vi "Manual Assembly old.vi"() -> ()   [LabVIEW 2021]
uses:
  Classes/Routine/Routine Enum.ctl
  Classes/Routine/TypeOfHexaboard.ctl
  Classes/Assembly/Assembly Run.lvclass
  Classes/Workspace/Fixture Enum.ctl
  Classes/Controller/Controller.lvclass
  Classes/Workspace/Fixture.lvclass
  Classes/Routine/Routine.lvclass
panel:
  in  "Submit":bool
  out "Type of Hexaboard Confirmation":T1
  in  "Type of Component":T1
  in  "Update":bool
  in  "Stage":i32(listbox)=-1
  in  "Routine":T2=enum."Dispense on Plate"
  in  "Stop":bool
  in  "Remove":bool
  in  "Add":bool
  in  "Go":bool
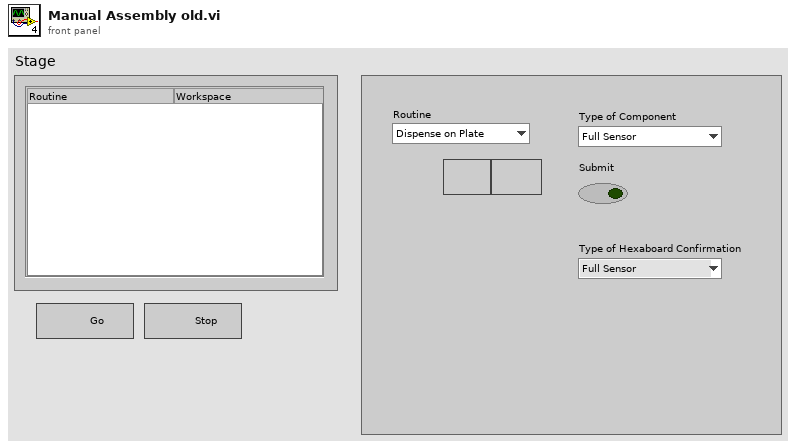
[diagram p1: front panel]
types:
  T1 = typedef "Routine.lvclass/TypeOfHexaboard.ctl" = enum16{"Full Sensor", "Full PCB", "Right Partial PCB", "Right Partial Sensor", "Al Dummy Right Partial Sensor"}
  T2 = typedef "Routine.lvclass/Routine Enum.ctl" = enum16{"Primary Pick Up", "Secondary Pick Up", "Put Down All", "Secure Syringe", "Release Syringe", "Dispense on Plate", "Dispense on Sensor", "Pick Up All", "Put Down Secondary", "Dispense on Kapton", "Full Assembly"}
  T3 = typedef "Controller.lvclass/Controllers.ctl" = cluster{"I-O.lvclass":refnum<class "I-O.lvclass">, "Gantry":refnum<k24>, "Dispenser":refnum<visa-resource-name>}
  T4 = typedef "Fixture.lvclass/Fixture Enum.ctl" = enum16{"Assembly Tray", "Syringe Space", "Component", "Pick Up Tool", "Current Position"}
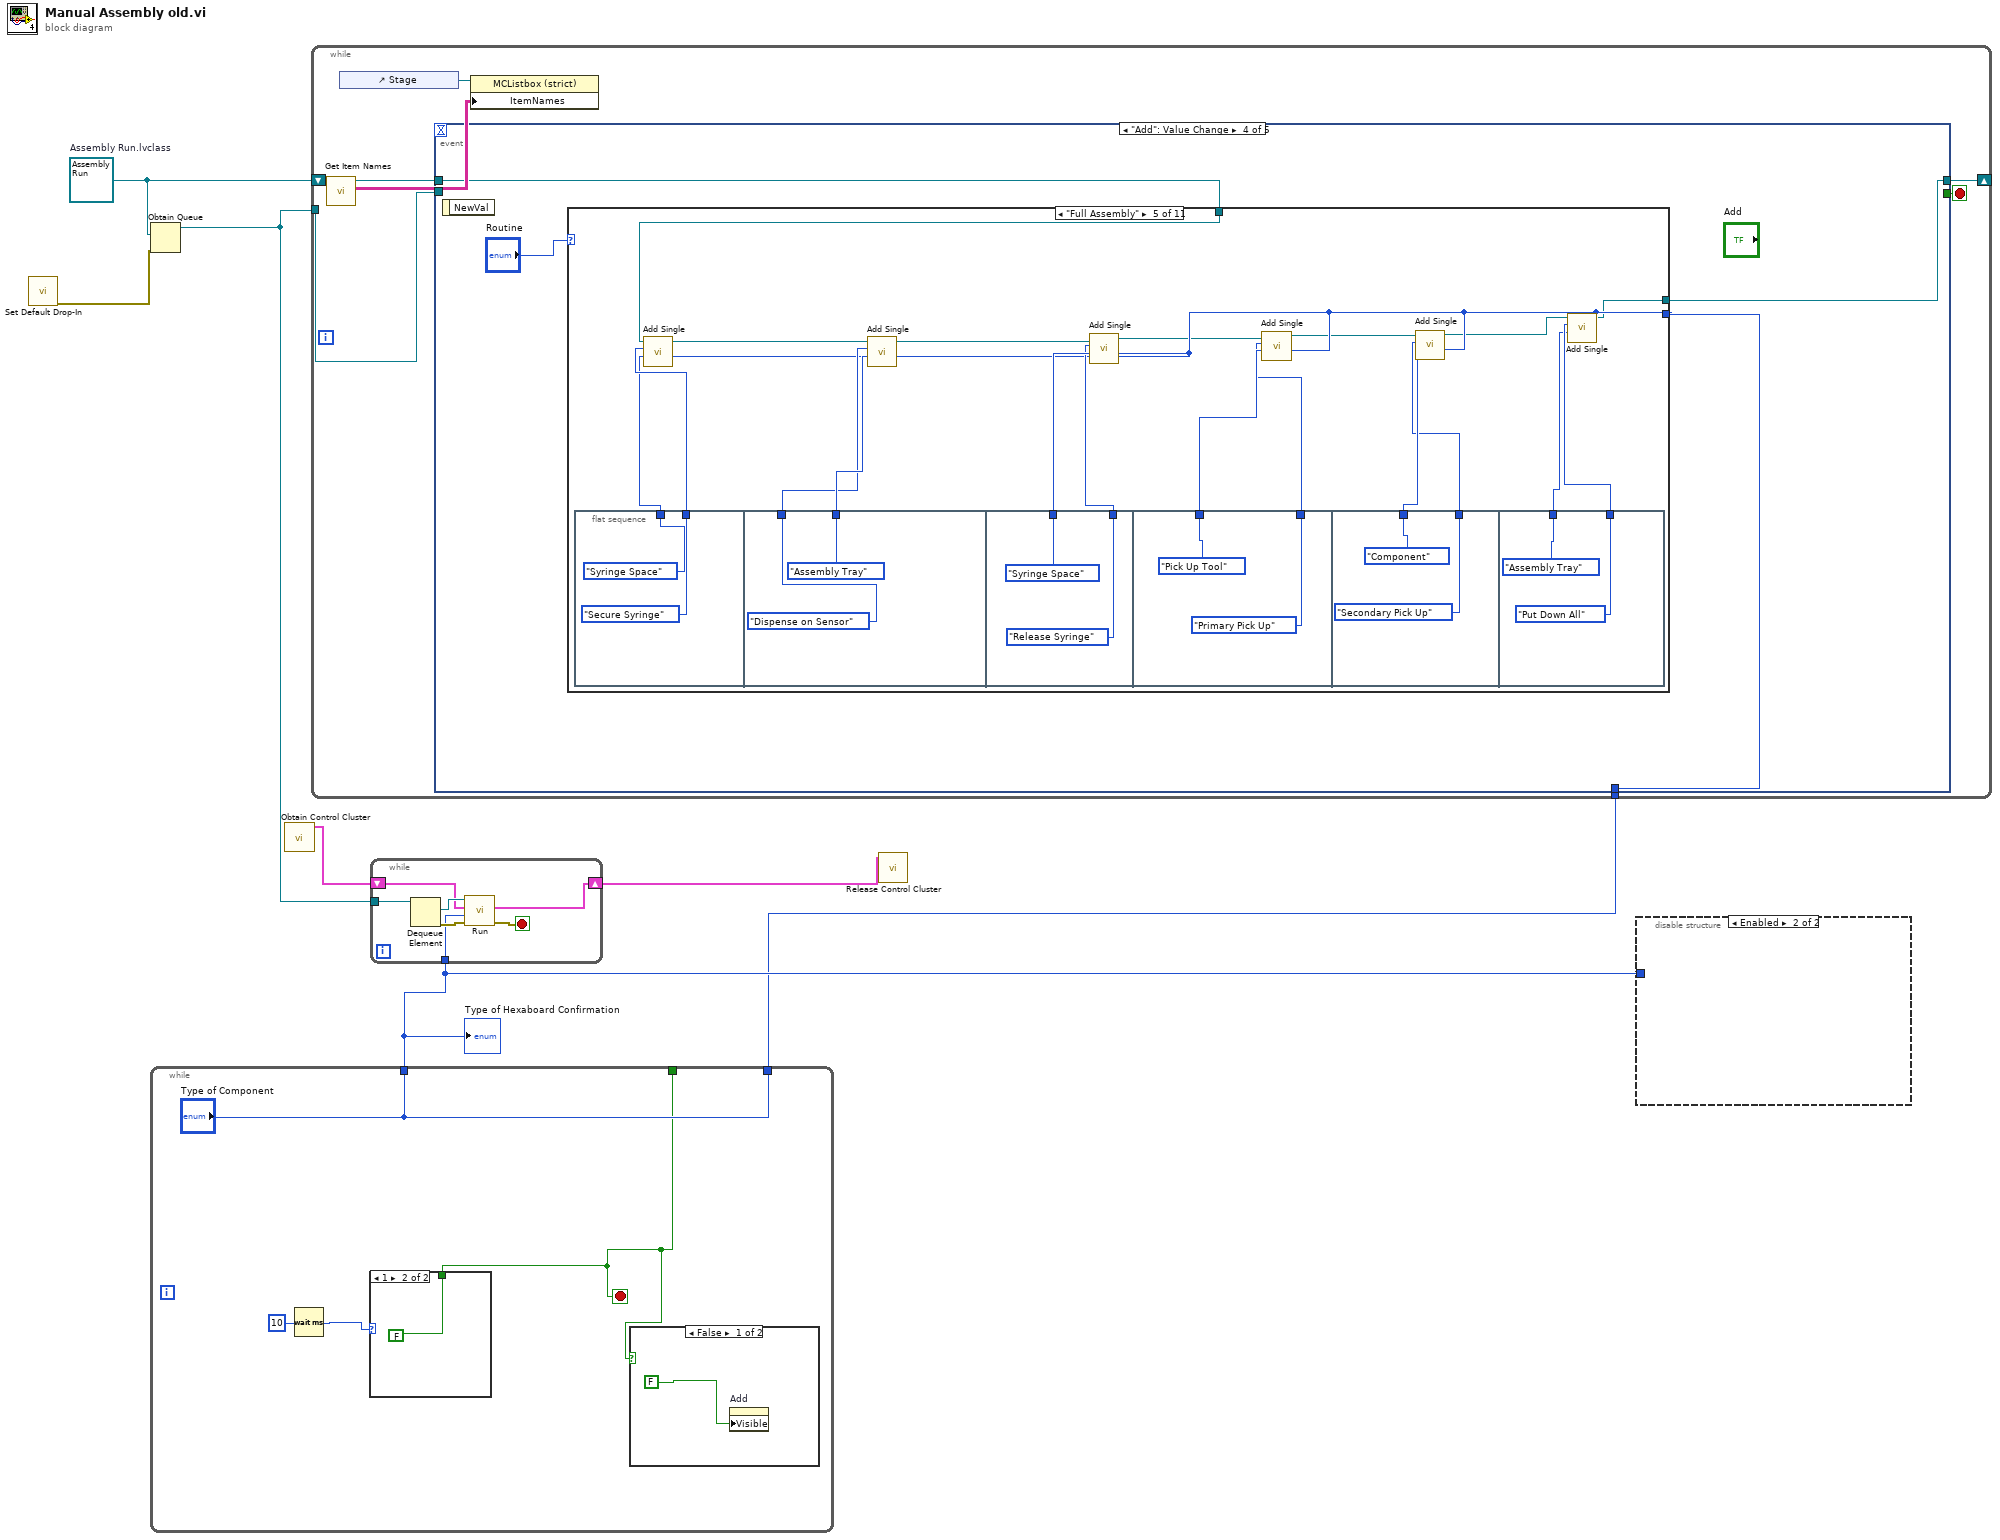
[diagram p0: block diagram]
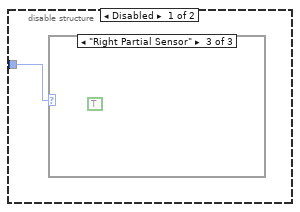
[diagram p2: hidden frame]
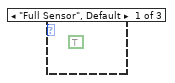
[diagram p3: hidden frame]
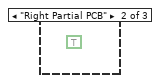
[diagram p4: hidden frame]
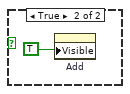
[diagram p5: hidden frame]
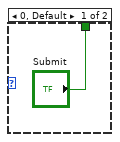
[diagram p6: hidden frame]
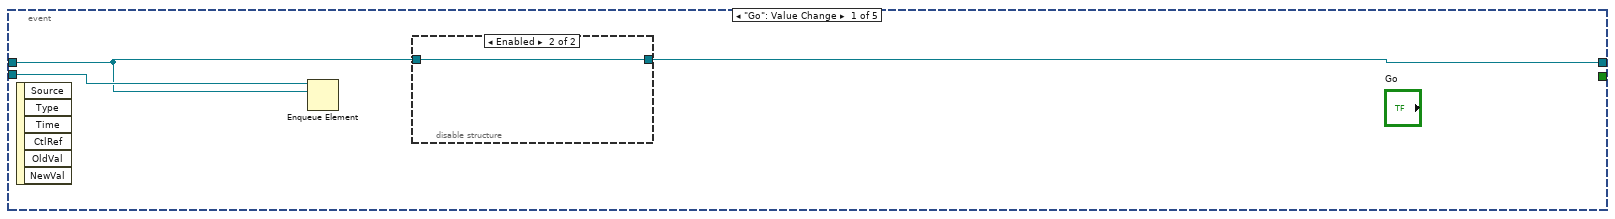
[diagram p7: hidden frame]
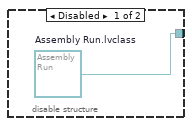
[diagram p8: hidden frame]
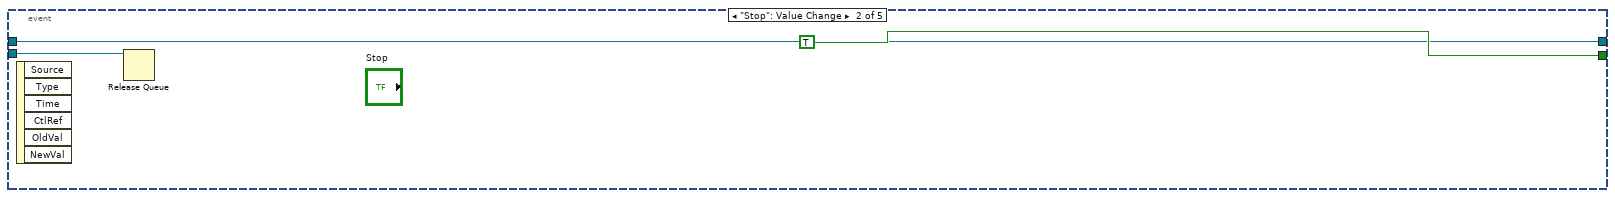
[diagram p9: hidden frame]
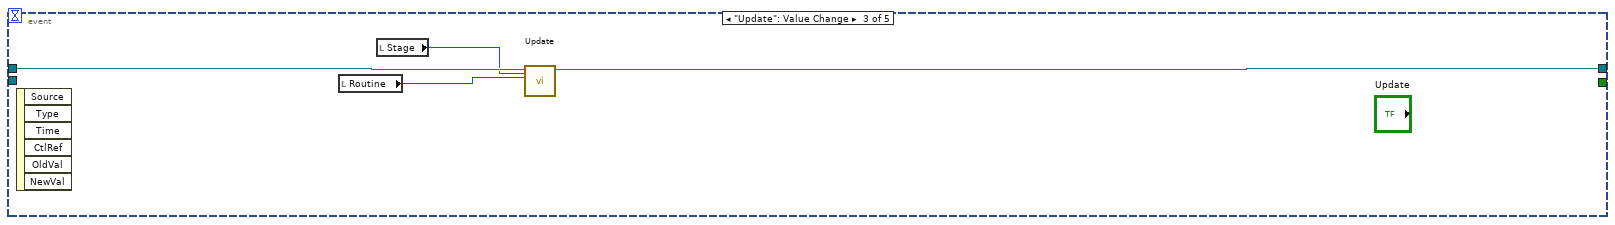
[diagram p10: hidden frame]
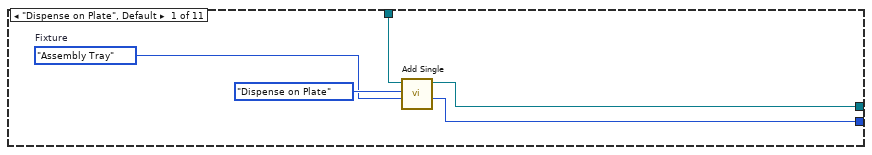
[diagram p11: hidden frame]
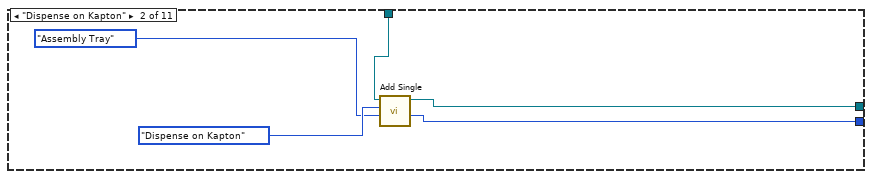
[diagram p12: hidden frame]
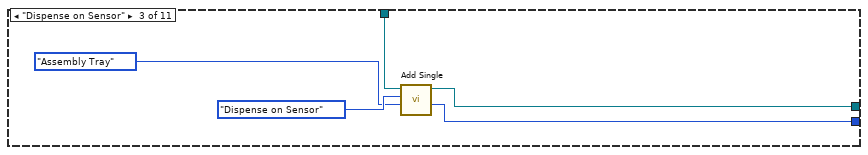
[diagram p13: hidden frame]
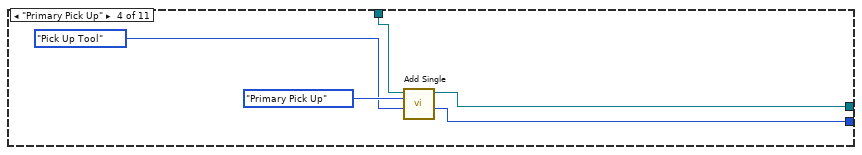
[diagram p14: hidden frame]
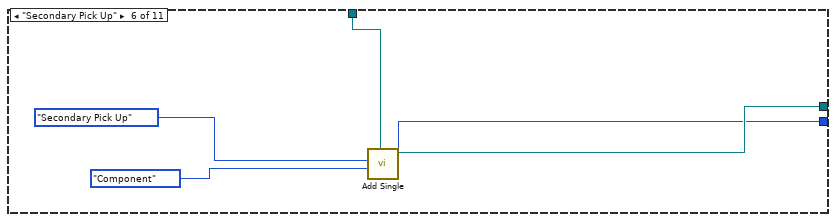
[diagram p15: hidden frame]
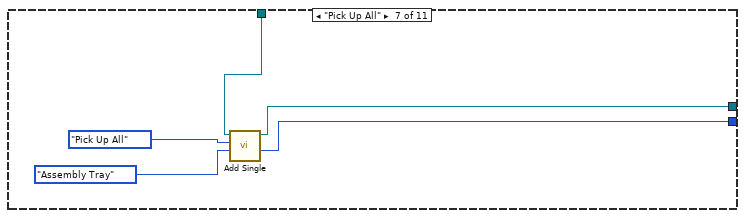
[diagram p16: hidden frame]
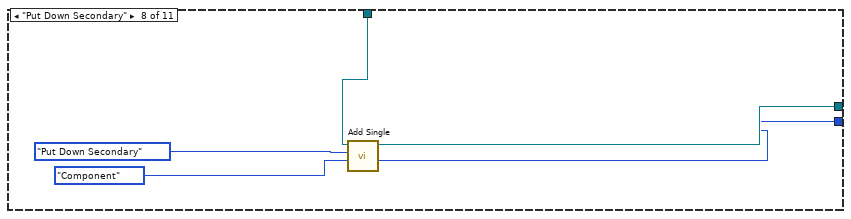
[diagram p17: hidden frame]
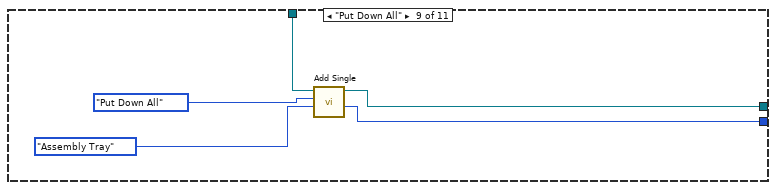
[diagram p18: hidden frame]
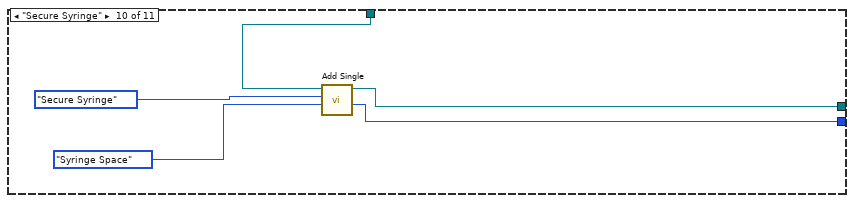
[diagram p19: hidden frame]
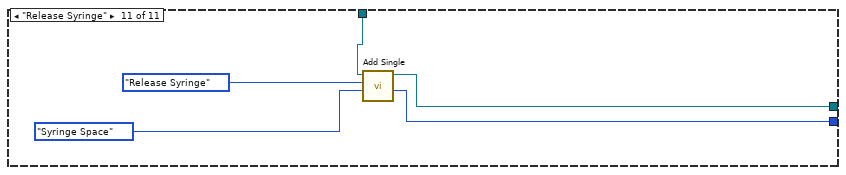
[diagram p20: hidden frame]
diagram:
  w3 = refnum<class "Assembly Run.lvclass"> refnum  # Assembly Run.lvclass
  n1 = call "Set Default Drop-In.vi"() -> ("error out"=w5:errorcluster)  [unwired: 11 in]
  n2 = Obtain Queue(element data type=w3, error in (no error)=w5) -> (queue out=w7:refnum<queue>)  [unwired: 3 in, 2 out]
  n3 = while {
    tunnel: ["Type of Component"] -> w2
    tunnel: ["Type of Component"] -> w1
    tunnel: [w8] -> _
    stop <- w8 stop-if-true
    n4 = Wait (ms)(milliseconds to wait=u32 10) -> (millisecond timer value=w10:u32)
    n5 = case shown="1" w10 {
      tunnel: ["Submit" FALSE] -> w8
      frame 0, Default {
      }
      frame 1 {
      }
    }
    n6 = case shown="False" w8 {
      frame False {
        n7 = property on="Add" class="Bool"("Visible"=FALSE) -> ()  [unwired: 2 in, 2 out]
      }
      frame True {
        n8 = property on="Add" class="Bool"("Visible"=TRUE) -> ()  [unwired: 2 in, 2 out]
      }
    }
  }
  "Type of Hexaboard Confirmation" <- w2
  n9 = call "Obtain Control Cluster.vi"() -> ("Control Out"=w4:T3)  [unwired: 11 in]
  n10 = while {
    shift-right: [w17] -> _
    shift-left: w3 -> [w19]
    tunnel: w7 -> [w22]
    tunnel: w1 -> [w16]
    stop <- w23 stop-if-true
    n11 = call "Get Item Names.vi"("Assembly Run in"=w19) -> ("Item names"=w21:string[][], "Assembly Run out"=w18:refnum<class "Assembly Run.lvclass">)  [unwired: 8 in, 1 out]
    n12 = control-ref of="Stage"() -> (w20:refnum<vi>)
    n13 = event shown="[3] \"Add\": Value Change" {
      selector: _ -> [_ _ _ _ _]
      dyn-events: _ -> [_ _ _ _ _]
      timeout: _ -> [_ _ _ _ _]
      tunnel: [_ TRUE _ _ _] -> w23
      tunnel: w18 -> [w24 w30 w35 w37 w124]
      tunnel: [w25 w30 w34 w36 w123] -> w17
      tunnel: w22 -> [w26 w29 _ _ _]
      tunnel: w16 -> [_ _ _ w38 _]
      event "Go": Value Change {
        n14 = event-data() -> ()  [unwired: 1 in, 6 out]
        n15 = Enqueue Element(queue=w26, element=w24) -> ()  [unwired: 2 in, 3 out]
        n16 = disable-structure shown="Enabled" {
          disable-tunnel: [w27 w28] -> w25
          disable-tunnel: w24 -> [_ w28]
          frame Disabled {
            w27 = refnum<class "Assembly Run.lvclass"> refnum  # Assembly Run.lvclass
          }
          frame Enabled {
          }
        }
      }
      event "Stop": Value Change {
        n17 = event-data() -> ()  [unwired: 1 in, 6 out]
        n18 = Release Queue(queue=w29) -> ()  [unwired: 2 in, 3 out]
      }
      event "Update": Value Change {
        n19 = event-data() -> ()  [unwired: 1 in, 6 out]
        n20 = local read "Routine"() -> (w33:T2)
        n21 = local read "Stage"() -> (w32:i32)
        n22 = call "Update.vi"("Row"=w32, "Routine"=w33, "Assembly Run in"=w35) -> ("Assembly Run out"=w34:refnum<class "Assembly Run.lvclass">)  [unwired: 7 in, 1 out]
      }
      event "Add": Value Change {
        n23 = event-data() -> ()  [unwired: 1 in, 1 out]
        n24 = case shown="\"Full Assembly\"" "Routine" {
          tunnel: w38 -> [w40 w47 w50 w55 w66 w92 w99 w102 w109 w114 w119]
          tunnel: w37 -> [w42 w45 w52 w56 w77 w94 w97 w103 w107 w112 w117]
          tunnel: [w41 w46 w51 w57 w60 w93 w98 w106 w108 w113 w118] -> w36
          frame "Dispense on Plate", Default {
            w43 = Fixture_Enum."Assembly Tray"  # Fixture
            n25 = call-dynamic "Add Single.vi"("Type of Hexaboard"=w40, "Fixture"=w43, "Routine"=Routine_Enum."Dispense on Plate", "UI in"=w42) -> ("UI out"=w41:refnum<class "Assembly Run.lvclass">)  [unwired: 5 in, 1 out]
          }
          frame "Dispense on Kapton" {
            n26 = call-dynamic "Add Single.vi"("Type of Hexaboard"=w47, "Fixture"=Fixture_Enum."Assembly Tray", "Routine"=Routine_Enum."Dispense on Kapton", "UI in"=w45) -> ("UI out"=w46:refnum<class "Assembly Run.lvclass">)  [unwired: 5 in, 1 out]
          }
          frame "Dispense on Sensor" {
            n27 = call-dynamic "Add Single.vi"("Type of Hexaboard"=w50, "Fixture"=Fixture_Enum."Assembly Tray", "Routine"=Routine_Enum."Dispense on Sensor", "UI in"=w52) -> ("UI out"=w51:refnum<class "Assembly Run.lvclass">)  [unwired: 5 in, 1 out]
          }
          frame "Primary Pick Up" {
            n28 = call-dynamic "Add Single.vi"("Type of Hexaboard"=w55, "Fixture"=Fixture_Enum."Pick Up Tool", "Routine"=Routine_Enum."Primary Pick Up", "UI in"=w56) -> ("UI out"=w57:refnum<class "Assembly Run.lvclass">)  [unwired: 5 in, 1 out]
          }
          frame "Full Assembly" {
            n29 = flat-sequence {
              tunnel: [Routine_Enum."Secure Syringe" ("Routine")] -> w79
              tunnel: [Fixture_Enum."Syringe Space" ("Fixture")] -> w78
              tunnel: [Fixture_Enum."Assembly Tray" ("Fixture")] -> w75
              tunnel: [Routine_Enum."Dispense on Sensor" ("Routine")] -> w74
              tunnel: [Fixture_Enum."Syringe Space" ("Fixture")] -> w73
              tunnel: [Routine_Enum."Release Syringe" ("Routine")] -> w72
              tunnel: [Fixture_Enum."Pick Up Tool" ("Fixture")] -> w71
              tunnel: [Routine_Enum."Primary Pick Up" ("Routine")] -> w70
              tunnel: [Fixture_Enum."Component" ("Fixture")] -> w69
              tunnel: [Routine_Enum."Secondary Pick Up" ("Routine")] -> w68
              tunnel: [Routine_Enum."Put Down All" ("Routine")] -> w67
              tunnel: [Fixture_Enum."Assembly Tray" ("Fixture")] -> w65
              frame #0 {
              }
              frame #1 {
              }
              frame #2 {
              }
              frame #3 {
              }
              frame #4 {
              }
              frame #5 {
              }
            }
            n30 = call-dynamic "Add Single.vi"("Type of Hexaboard"=w66, "Fixture"=w78, "Routine"=w79, "UI in"=w77) -> ("UI out"=w76:refnum<class "Assembly Run.lvclass">)  [unwired: 5 in, 1 out]
            n31 = call-dynamic "Add Single.vi"("Type of Hexaboard"=w66, "Fixture"=w75, "Routine"=w74, "UI in"=w76) -> ("UI out"=w64:refnum<class "Assembly Run.lvclass">)  [unwired: 5 in, 1 out]
            n32 = call-dynamic "Add Single.vi"("Type of Hexaboard"=w66, "Fixture"=w73, "Routine"=w72, "UI in"=w64) -> ("UI out"=w63:refnum<class "Assembly Run.lvclass">)  [unwired: 5 in, 1 out]
            n33 = call-dynamic "Add Single.vi"("Type of Hexaboard"=w66, "Fixture"=w71, "Routine"=w70, "UI in"=w63) -> ("UI out"=w62:refnum<class "Assembly Run.lvclass">)  [unwired: 5 in, 1 out]
            n34 = call-dynamic "Add Single.vi"("Type of Hexaboard"=w66, "Fixture"=w69, "Routine"=w68, "UI in"=w62) -> ("UI out"=w61:refnum<class "Assembly Run.lvclass">)  [unwired: 5 in, 1 out]
            n35 = call-dynamic "Add Single.vi"("Type of Hexaboard"=w66, "Fixture"=w65, "Routine"=w67, "UI in"=w61) -> ("UI out"=w60:refnum<class "Assembly Run.lvclass">)  [unwired: 5 in, 1 out]
          }
          frame "Secondary Pick Up" {
            n36 = call-dynamic "Add Single.vi"("Type of Hexaboard"=w92, "Fixture"=Fixture_Enum."Component", "Routine"=Routine_Enum."Secondary Pick Up", "UI in"=w94) -> ("UI out"=w93:refnum<class "Assembly Run.lvclass">)  [unwired: 5 in, 1 out]
          }
          frame "Pick Up All" {
            n37 = call-dynamic "Add Single.vi"("Type of Hexaboard"=w99, "Fixture"=Fixture_Enum."Assembly Tray", "Routine"=Routine_Enum."Pick Up All", "UI in"=w97) -> ("UI out"=w98:refnum<class "Assembly Run.lvclass">)  [unwired: 5 in, 1 out]
          }
          frame "Put Down Secondary" {
            n38 = call-dynamic "Add Single.vi"("Type of Hexaboard"=w102, "Fixture"=Fixture_Enum."Component", "Routine"=Routine_Enum."Put Down Secondary", "UI in"=w103) -> ("UI out"=w106:refnum<class "Assembly Run.lvclass">)  [unwired: 5 in, 1 out]
          }
          frame "Put Down All" {
            n39 = call-dynamic "Add Single.vi"("Type of Hexaboard"=w109, "Fixture"=Fixture_Enum."Assembly Tray", "Routine"=Routine_Enum."Put Down All", "UI in"=w107) -> ("UI out"=w108:refnum<class "Assembly Run.lvclass">)  [unwired: 5 in, 1 out]
          }
          frame "Secure Syringe" {
            n40 = call-dynamic "Add Single.vi"("Type of Hexaboard"=w114, "Fixture"=Fixture_Enum."Syringe Space", "Routine"=Routine_Enum."Secure Syringe", "UI in"=w112) -> ("UI out"=w113:refnum<class "Assembly Run.lvclass">)  [unwired: 5 in, 1 out]
          }
          frame "Release Syringe" {
            n41 = call-dynamic "Add Single.vi"("Type of Hexaboard"=w119, "Fixture"=Fixture_Enum."Syringe Space", "Routine"=Routine_Enum."Release Syringe", "UI in"=w117) -> ("UI out"=w118:refnum<class "Assembly Run.lvclass">)  [unwired: 5 in, 1 out]
          }
        }
      }
      event "Remove": Value Change {
        n42 = event-data() -> ()  [unwired: 1 in, 6 out]
        n43 = call "Delete.vi"("Index"="Stage", "Assembly In"=w124) -> ("Assembly Out"=w123:refnum<class "Assembly Run.lvclass">)  [unwired: 8 in, 1 out]
      }
    }
    n44 = property class="MCListbox (strict)"(reference=w20, "ItemNames"=w21) -> ()  [unwired: 1 in, 2 out]
  }
  n45 = while {
    tunnel: w7 -> [w131]
    shift-right: [w126] -> w6
    shift-left: w4 -> [w127]
    tunnel: w2 -> [w125]
    stop <- w128 stop-if-true
    n46 = Dequeue Element(queue=w131) -> (element=w130:refnum<class "Assembly Run.lvclass">, error out=w129:errorcluster)  [unwired: 2 in, 2 out]
    n47 = call-dynamic "Run.vi"("error in (no error)"=w129, "Type of Hexaboard"=w125, "Control In"=w127, "Assembly In"=w130) -> ("error out"=w128:errorcluster, "Control Out"=w126:T3)  [unwired: 5 in, 1 out]
  }
  n48 = call "Release Control Cluster.vi"("output cluster"=w6) -> ()  [unwired: 11 in]
  n49 = disable-structure shown="Enabled" {
    disable-tunnel: w2 -> [w132 _]
    frame Disabled {
      n50 = case shown="\"Right Partial Sensor\"" w132 {
        frame "Full Sensor", Default {
          w133 = TRUE
        }
        frame "Right Partial PCB" {
          w134 = TRUE
        }
        frame "Right Partial Sensor" {
          w135 = TRUE
        }
      }
    }
    frame Enabled {
    }
  }
